vi "Test ReadDevicePlatform.vi"() -> ()   [LabVIEW 2020]
uses:
  VisaResource/VisaResource.lvclass
  C:/dev/Vireo/PicoG/PicoG-Processor/PicoG-Core/DeployResource/DeployResource.lvclass
  DeployResource/DeployResource.lvclass
panel:
  out "error out":errorcluster
  out "Platform":string
  in  "Resource":refnum<visa-resource-name>
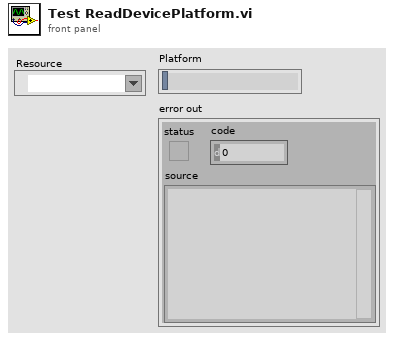
[diagram p1: front panel]
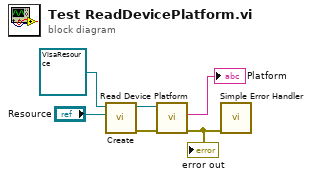
[diagram p0: block diagram]
diagram:
  n1 = call-dynamic "Create.vi"("Resource"="Resource", "VisaResource in"=refnum<class "VisaResource.lvclass"> refnum) -> ("error out"=w4:errorcluster, "VisaResource out"=w3:refnum<class "VisaResource.lvclass">)  [unwired: 8 in]
  n2 = call "Read Device Platform.vi"("error in (no error)"=w4, "Resource in"=w3) -> ("error out"=w1:errorcluster, "Platform"=→"Platform":string)  [unwired: 7 in, 1 out]
  "error out" <- w1
  n3 = call <vilib>:"Simple Error Handler.vi"("error in (no error)"=w1) -> ()  [unwired: 4 in, 5 out]
